vi "Class polymorphism Example.vi"() -> ()   [LabVIEW 2014]
doc: "Shows how to do general polymorphims. Two children classes, different return string, but interface is the same --> parent class with exactly defined methods common for all children classes."
uses:
  utils/PointerInt32Datatype.lvclass
  utils/PointerDatatype.lvclass
  utils/PointerStringDatatype.lvclass
panel:
  out "datatype 2":string="void*"
  out "datatype":string="void*"
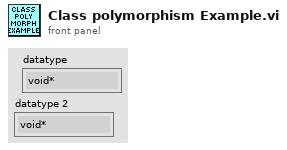
[diagram p1: front panel]
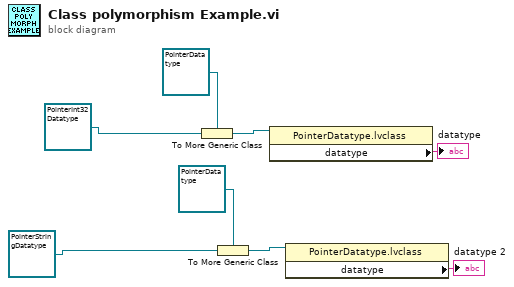
[diagram p0: block diagram]
diagram:
  n1 = To More Generic Class(target class=refnum<class "PointerDatatype.lvclass"> refnum ("PointerDatatype.lvclass"), reference=refnum<class "PointerInt32Datatype.lvclass"> refnum ("PointerInt32Datatype.lvclass")) -> (generic class reference=w6:refnum<class "PointerDatatype.lvclass">)
  n2 = To More Generic Class(target class=refnum<class "PointerDatatype.lvclass"> refnum ("PointerDatatype.lvclass"), reference=refnum<class "PointerStringDatatype.lvclass"> refnum ("PointerStringDatatype.lvclass")) -> (generic class reference=w4:refnum<class "PointerDatatype.lvclass">)
  n3 = property class="PointerDatatype.lvclass"(reference=w6) -> ("datatype"=→"datatype":string)  [unwired: 1 in, 2 out]
  n4 = property class="PointerDatatype.lvclass"(reference=w4) -> ("datatype"=→"datatype 2":string)  [unwired: 1 in, 2 out]
